vi "Set Wheel Radius.vi"(7 "generate error if invalid (T)":bool=TRUE, 8 "error in (no error)":errorcluster, 10 "wheel radius":dbl, 11 "wheel in":refnum<class "NI_Robotics_Wheel.lvclass">) -> (0 "error out":errorcluster, 1 "valid?":bool, 3 "wheel out":refnum<class "NI_Robotics_Wheel.lvclass">)   [LabVIEW 2017, in "NI_Robotics_Wheel.lvclass"]
uses:
  <vilib>/robotics/Steering/Wheel/NI_Robotics_Wheel.lvclass
  <vilib>/robotics/Steering/Wheel/NI_Robotics_Wheel.lvclass/NI_Robotics_Wheel.ctl
  <vilib>/robotics/Utilities/NI_Robotics Utilities.lvlib
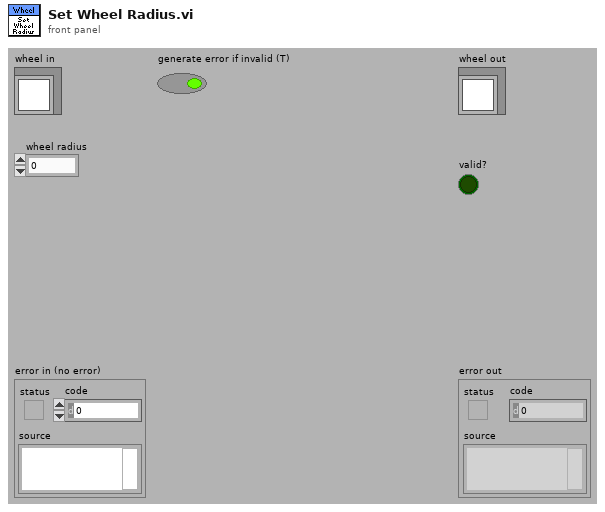
[diagram p1: front panel]
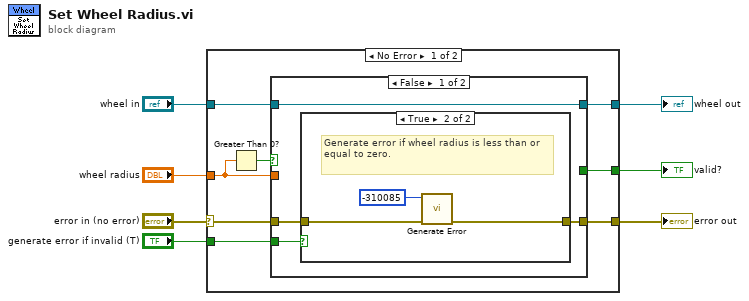
[diagram p0: block diagram]
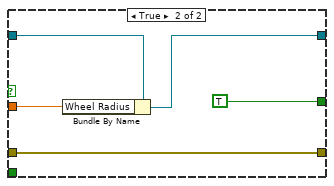
[diagram p3: hidden frame]
diagram:
  n1 = case shown="No Error" "error in (no error)" {
    selector: "error in (no error)" -> [w11 w29]
    tunnel: [w10 w29] -> w6
    tunnel: [w14 w30] -> w4
    tunnel: "wheel in" -> [w15 w30]
    tunnel: "wheel radius" -> [w13 _]
    tunnel: "generate error if invalid (T)" -> [w9 _]
    tunnel: [w8 _] -> w1
    frame No Error {
      n2 = Greater Than 0?(x=w13) -> (x > 0?=w12:bool)
      n3 = case shown="False" w12 {
        tunnel: w15 -> [w17 w28]
        tunnel: [w17 w27] -> w14
        tunnel: w13 -> [_ w26]
        tunnel: w11 -> [w19 w25]
        tunnel: [w18 w25] -> w10
        tunnel: w9 -> [w16 _]
        tunnel: [_ TRUE] -> w8
        frame False {
          n4 = case shown="True" w16 {
            tunnel: w19 -> [w20 w22]
            tunnel: [w20 w21] -> w18
            frame False {
            }
            frame True {
              # "Generate error if wheel radius is less than or equal to zero."
              n5 = call <vilib>:"Generate Error.vi"("error in (no error)"=w22, "code"=-310085 ("chain levels to remove (1)")) -> ("error out"=w21:errorcluster)  [unwired: 9 in]
            }
          }
        }
        frame True {
          n6 = Bundle By Name(cluster=w28, "Wheel Radius"=w26) -> (w27:refnum<class "NI_Robotics_Wheel.lvclass">)
        }
      }
    }
    frame Error {
    }
  }
  "error out" <- w6
  "wheel out" <- w4
  "valid?" <- w1
